vi "Get Event Log.vi"(8 "error in (no error)":errorcluster, 10 "Log Type (0: All Event Log)":i32(ring) items=["All Event Log", "Oldest Event Log"], 11 "VISA resource name":refnum<visa-resource-name>) -> (0 "error out":errorcluster, 1 "Log Count":i32, 2 "Log":string, 3 "VISA resource name out":refnum<visa-resource-name>)   [LabVIEW 2017, in "Keithley 2600 Series.lvlib"]
doc: "Returns the event log as a single string and removes them from the event log."
uses:
  <instrlib>/Keithley 2600 Series/Keithley 2600 Series.lvlib
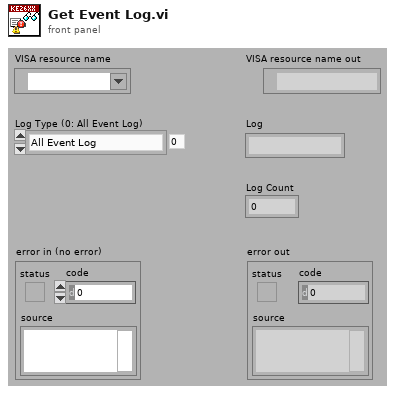
[diagram p1: front panel]
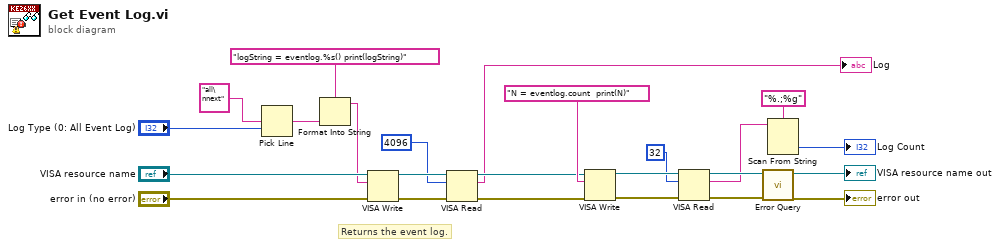
[diagram p0: block diagram]
diagram:
  # "Returns the event log."
  n1 = Pick Line(multi-line string="all\nnext", line index="Log Type (0: All Event Log)") -> (output string=w18:string)  [unwired: 1 in]
  n2 = Format Into String(format string="logString = eventlog.%s() print(logString)", w18) -> (resulting string=w16:string)  [unwired: 2 in, 1 out]
  n3 = VISA Write(VISA resource name="VISA resource name", write buffer=w16, error in (no error)="error in (no error)") -> (VISA resource name out=w15:refnum<visa-resource-name>, error out=w14:errorcluster)  [unwired: 1 out]
  n4 = VISA Read(VISA resource name=w15, byte count=u32 4096, error in (no error)=w14) -> (VISA resource name out=w9:refnum<visa-resource-name>, read buffer=→"Log":string, error out=w8:errorcluster)  [unwired: 1 out]
  n5 = VISA Write(VISA resource name=w9, write buffer="N = eventlog.count  print(N)", error in (no error)=w8) -> (VISA resource name out=w13:refnum<visa-resource-name>, error out=w12:errorcluster)  [unwired: 1 out]
  n6 = VISA Read(VISA resource name=w13, byte count=u32 32, error in (no error)=w12) -> (VISA resource name out=w6:refnum<visa-resource-name>, read buffer=w2:string, error out=w5:errorcluster)  [unwired: 1 out]
  n7 = call <instrlib>:"Error Query.vi"("error in (no error)"=w5, "VISA resource name"=w6) -> ("error out"=→"error out":errorcluster, "VISA resource name out"=→"VISA resource name out":refnum<visa-resource-name>)  [unwired: 6 in, 2 out]
  n8 = Scan From String(format string="%.;%g", input string=w2) -> (output 1=→"Log Count":i32)  [unwired: 3 in, 3 out]
